vi "Experiment_Settings_Live.vi"() -> ()   [LabVIEW 2013]
uses:
  Public API/DisplayExperimentSetting.ctl
panel:
  in  "stop":bool
  in  "small?":bool
  out "error out":errorcluster
  in  "error in (no error)":errorcluster
  out "Experiment Settings":T1
  # "Experiment Status:"
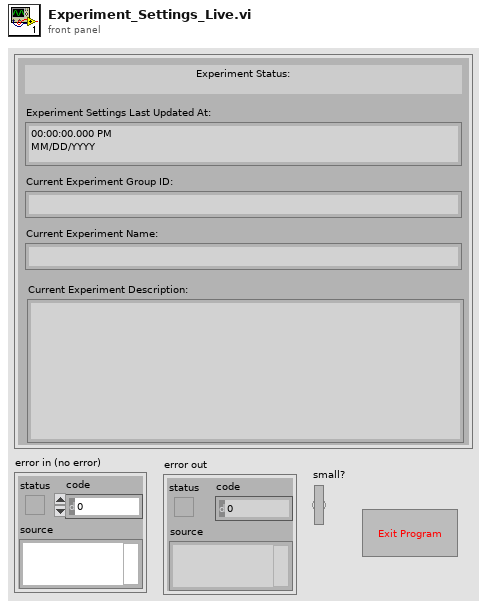
[diagram p1: front panel]
types:
  T1 = typedef "DisplayExperimentSetting.ctl" = cluster{"Current Experiment Name:":string, "Current Experiment Description:":string, "Current Experiment Group ID:":string, "Experiment Settings Last Updated At:":timestamp}
  T2 = typedef "LVRectTypeDef.ctl" = cluster{"Left":i16, "Top":i16, "Right":i16, "Bottom":i16}
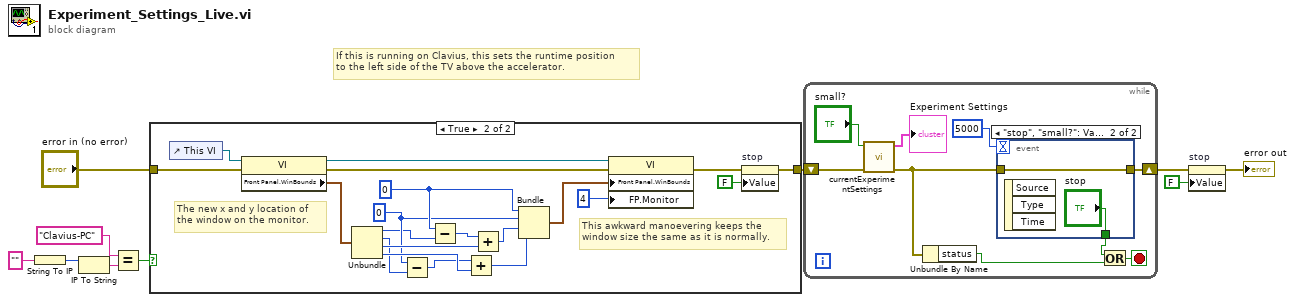
[diagram p0: block diagram]
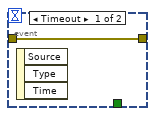
[diagram p3: hidden frame]
diagram:
  # "If this is running on Clavius, this sets the runtime position\nto the left side of the TV above the accelerator."
  n1 = String To IP(1:"" ("name")) -> (0:w7:u32)
  n2 = IP To String(2:w7) -> (0:w9:string)  [unwired: 1 in]
  n3 = Equal?(x="Clavius-PC", y=w9) -> (x = y?=w5:bool)
  n4 = case shown="True" w5 {
    tunnel: "error in (no error)" -> [w11 w16]
    tunnel: [w11 w13] -> w4
    frame False {
    }
    frame True {
      w21 = i16 0 ("Top")
      w22 = i16 0 ("Left")
      # "This awkward manoevering keeps the\nwindow size the same as it is normally."
      # "The new x and y location of\nthe window on the monitor."
      n5 = control-ref of="This VI"() -> (w30:refnum<vi>)
      n6 = property class="VI"(reference=w30, error in=w16) -> (reference out=w26:refnum<vi>, error out=w15:errorcluster, "Front Panel.WinBounds"=w25:T2)
      n7 = Unbundle(w25) -> ("Left"=w20:i16, "Top"=w19:i16, "Right"=w24:i16, "Bottom"=w23:i16)
      n8 = Subtract(x=w21, y=w19) -> (x-y=w18:i16)
      n9 = Subtract(x=w22, y=w20) -> (x-y=w17:i16)
      n10 = Add(x=w18, y=w23) -> (x+y=w27:i16)
      n11 = Add(x=w17, y=w24) -> (x+y=w28:i16)
      n12 = Bundle("Left"=w22, "Top"=w21, w28, w27) -> (w31:cluster{"Left":i16, "Top":i16, i16, i16})  [unwired: 1 in]
      n13 = property class="VI"(reference=w26, error in=w15, "Front Panel.WinBounds"=w31, "FP.Monitor"=u16 4 ("Front Panel Window:Monitor")) -> (error out=w12:errorcluster)  [unwired: 1 out]
      n14 = property on="stop" class="Bool (strict)"(error in=w12, "Value"=FALSE ("stop")) -> (error out=w13:errorcluster)  [unwired: 1 in, 1 out]
    }
  }
  n15 = while {
    shift-right: [w40] -> w10
    shift-left: w4 -> [w38]
    stop <- w35 stop-if-true
    n16 = call "currentExperimentSettings.vi"("error in (no error)"=w38, "small?"="small?") -> ("error out"=w33:errorcluster, "output cluster"=→"Experiment Settings":T1)  [unwired: 4 in, 4 out]
    n17 = Unbundle By Name(w33) -> ("status"=w32:bool)
    n18 = event shown="[1] \"stop\", \"small?\": Value Change" {
      selector: _ -> [_ _]
      dyn-events: _ -> [_ _]
      timeout: u32 5000 ("milliseconds to wait") -> [_ _]
      tunnel: w33 -> [w41 w42]
      tunnel: [w41 w42] -> w40
      tunnel: [_ "stop"] -> w34
      event Timeout {
        n19 = event-data() -> ()  [unwired: 1 in, 3 out]
      }
      event "stop", "small?": Value Change {
        n20 = event-data() -> ()  [unwired: 1 in, 3 out]
      }
    }
    n21 = Or(x=w34, y=w32) -> (x .or. y?=w35:bool)
  }
  n22 = property on="stop" class="Bool (strict)"(error in=w10, "Value"=FALSE ("stop")) -> (error out=→"error out":errorcluster)  [unwired: 1 in, 1 out]
